vi "acquisitionGetFrame8bit.vi"(1 "resize":bool, 2 "index":i32, 3 "hamamatsuFrameReferences":refnum<data-value>[](array[refnum])) -> (0 "frameOut":u8[][](array[numeric]))   [LabVIEW 2017]
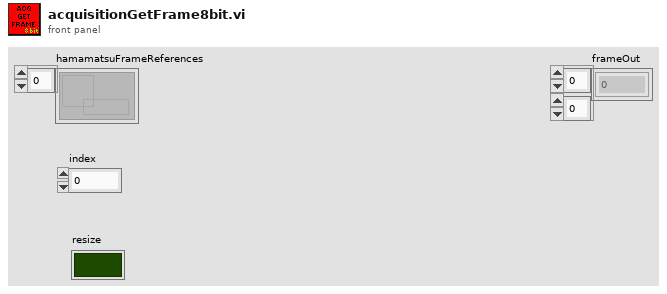
[diagram p1: front panel]
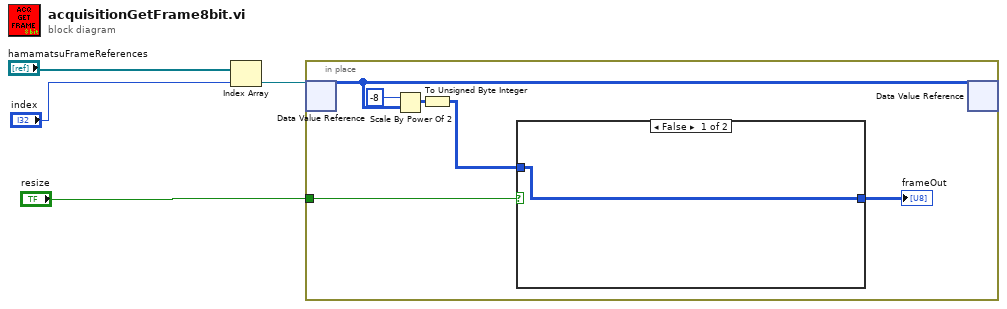
[diagram p0: block diagram]
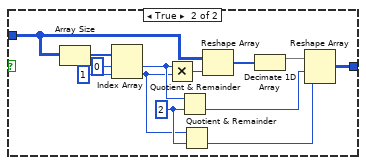
[diagram p2: hidden frame]
diagram:
  n1 = Index Array(array="hamamatsuFrameReferences", index="index") -> (element=w2:refnum<data-value>)
  n2 = in-place {
    in-place-border: "resize" -> [w6]
    n3 = in-place-dvr #1(w2) -> (w10:u16[][])  [unwired: 1 out]
    n4 = Scale By Power Of 2(n=i16 -8, x=w10) -> (x*2^n=w8:u16[][])
    n5 = To Unsigned Byte Integer(number=w8) -> (unsigned 8bit integer=w7:u8[][])
    n6 = case shown="False" w6 {
      tunnel: w7 -> [w11 w19]
      tunnel: [w11 w12] -> w5
      frame False {
      }
      frame True {
        w17 = 2 ("y")
        n7 = Array Size(array=w19) -> (size(s)=w24:i32[])
        n8 = Index Array(array=w24, index #1=0 ("index"), index #2=1 ("index")) -> (element #1=w18:i32, element #2=w16:i32)
        n9 = Multiply(x=w18, y=w16) -> (x*y=w21:i32)
        n10 = Quotient & Remainder(x=w18, y=w17) -> (floor(x/y)=w14:i32)  [unwired: 1 out]
        n11 = Quotient & Remainder(x=w16, y=w17) -> (floor(x/y)=w13:i32)  [unwired: 1 out]
        n12 = Reshape Array(w19, w21) -> (w20:u8[])
        n13 = Decimate 1D Array(w20) -> (w15:u8[])  [unwired: 1 out]
        n14 = Reshape Array(w15, w14, w13) -> (w12:u8[][])
      }
    }
    "frameOut" <- w5
    n15 = in-place-dvr #1(w10) -> ()  [unwired: 2 out]
  }
